vi "DepthSense Verbose Acquisition.vi"() -> ()   [LabVIEW 2011]
uses:
  <vilib>/vision/Image Controls.llb/IMAQ Image.ctl
  <vilib>/Platform/TimedLoop/XDataNode/timing_clust.ctl
  <vilib>/Platform/TimedLoop/XDataNode/nitl_modes.ctl
  <vilib>/Platform/TimedLoop/XDataNode/wakeup.ctl
  C:/Users/Behavior Room/Desktop/Kinect Mouse/DepthSense/FunctionPointerProxy/FunctionPointerProxy/bin/Release/FunctionPointerProxy.dll
  FunctionPointerProxy/FunctionPointerProxy/bin/Release/FunctionPointerProxy.dll
  IT WORKS SO SUCK IT/DepthSense Global Status.vi
  <vilib>/Platform/TimedLoop/XDataNode/XDataNode.xnode
  <userlib>/libOptrima-2-3/libOptrima-2-3.lvlib
  <vilib>/Platform/TimedLoop/XDataNode/XDNodeRunTimeDep.lvlib
  Program Files (x86)/SoftKinetic/OptrimaSDK/lib/libOptrima-2-3.dll
panel:
  out "Image":T1(plugin-control)
  out "Frame ID":i32
  in  "DepthSense Indicator":T2={"Camera Version"="", "Image Height"=0, "Image Width"=0, "Minimum Framerate"=0, "Maximum Framerate"=0, "Framerate"=25, "Close Mode"=FALSE, "Denoising"=FALSE, "Leakage Algorithm"=FALSE, "Anti-Aliasing"=FALSE, "Camera Status"=-2, "API Version"="", "Light Intensity"=100, "Confidence Threshold"=100, "Range"=0.0}
  in  "stop":bool
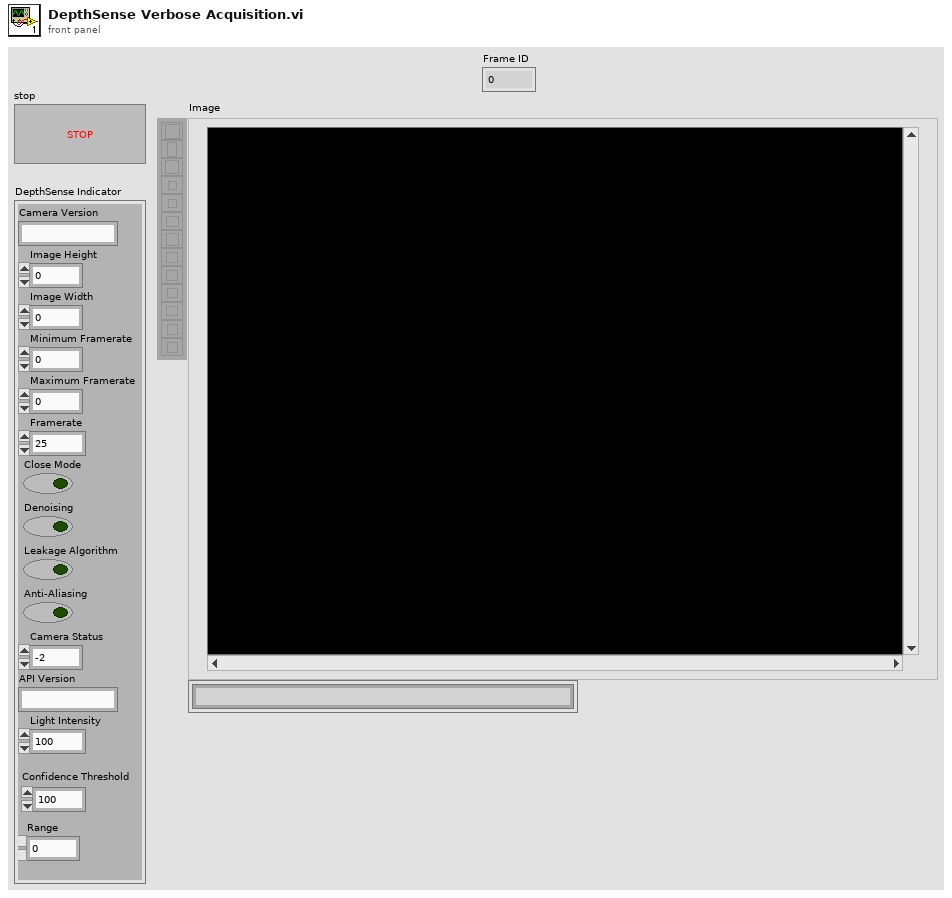
[diagram p1: front panel]
types:
  T1 = typedef "IMAQ Image.ctl" = refnum<image>
  T2 = cluster{"Camera Version":string, "Image Height":i32, "Image Width":i32, "Minimum Framerate":i32, "Maximum Framerate":i32, "Framerate":i32, "Close Mode":bool, "Denoising":bool, "Leakage Algorithm":bool, "Anti-Aliasing":bool, "Camera Status":i32, "API Version":string, "Light Intensity":i32, "Confidence Threshold":u16, "Range":dbl}
  T3 = cluster{"Camera Version":string, "Image Height":i32, "Image Width":i32, "Minimum Framerate":i32, "Maximum Framerate":i32, "Framerate":i32, "Close Mode":bool, "Denoising":bool, "Leakage Algorithm":bool, "Anti-Aliasing":bool, "Camera Status":i32, "API Version":string, "Light Intensity":i32, "Confidence Threshold":u16, "Range":sgl}
  T4 = typedef "t_CallbackReferences.ctl" = cluster{"LV event callback ":refnum<k27>, "Proxy instance":refnum<k24>, "(*f)(...)":i32}
  T5 = typedef "XDNodeRunTimeDep.lvlib/timing_clust.ctl" = cluster{"Expected End [f-1]":u64, "Actual End [f-1]":u64, "Finished Late? [f-1]":bool, "Expected End [i-1]":u64, "Actual End [i-1]":u64, "Finished Late? [i-1]":bool, "Expected Start [i]":u64, "Actual Start [i]":u64, "Expected Start [f]":u64, "Actual Start [f]":u64, "Source Name":string, "Structure Name":string, "Period":i64, "Deadline":i64, "Offset":i64, "Start":i64, "Priority":i32, "Timeout":i32, "Mode":T6, "Wakeup Reason":T7, "Error":errorcluster, "Source Type":string, "Secondary Source Type":string, "Global End Time":u64, "Global Start Time":u64, "Frame Duration":u64, "Iteration Duration":u64, "Assigned CPU":i32, "I/O Scan Engine Mode":u32}
  T6 = typedef "XDNodeRunTimeDep.lvlib/nitl_modes.ctl" = enum32{"No Change", "Process missed periods, maintain original phase", "Discard missed periods, maintain original phase", "Process missed periods, ignore original phase", "Discard missed periods, ignore original phase"}
  T7 = typedef "XDNodeRunTimeDep.lvlib/wakeup.ctl" = enum32{"Normal", "Aborted", "Asynchronous wakeup", "Timing source error", "Timed loop error", "Timeout"}
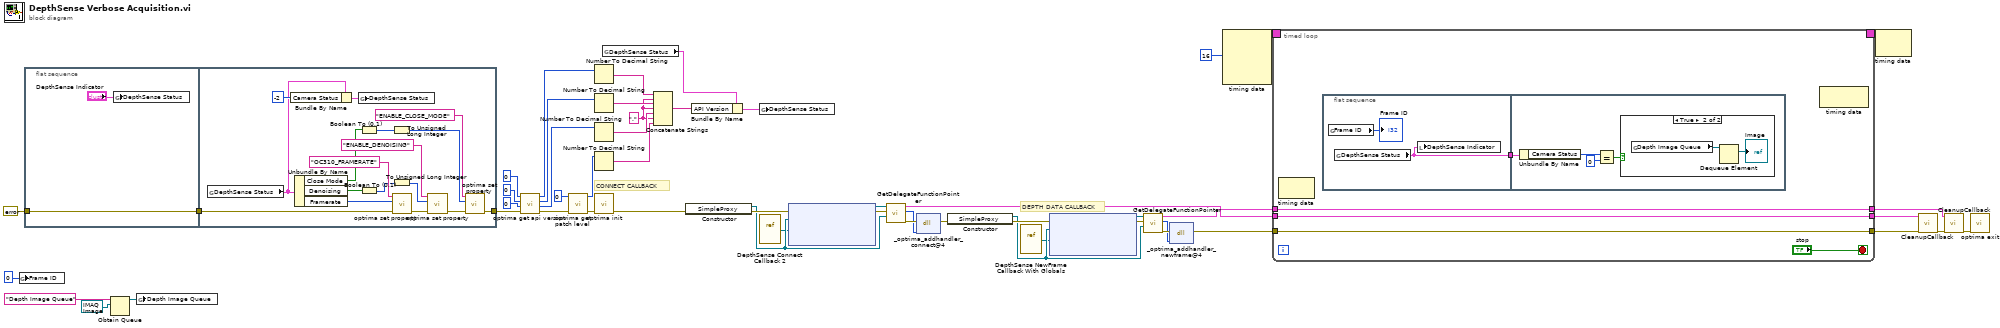
[diagram p0: block diagram]
diagram:
  w39 = "."
  # "DEPTH DATA CALLBACK"
  # "CONNECT CALLBACK"
  n1 = global write "DepthSense Global Status.vi" "Frame ID"(0 ("Frame ID")) -> ()
  n2 = flat-sequence {
    tunnel: errorcluster {"status"=FALSE, "code"=0, "source"=""} ("error in (no error)") -> [w54]
    tunnel: [w54] -> w1
    tunnel: [w69] -> w9
    tunnel: w1 -> [w63]
    frame #0 {
      n3 = global write "DepthSense Global Status.vi" "DepthSense Status"("DepthSense Indicator") -> ()
    }
    frame #1 {
      n4 = global read "DepthSense Global Status.vi" "DepthSense Status"() -> (w62:T3)
      n5 = Bundle By Name(cluster=w62, "Camera Status"=-2) -> (w71:T3)
      n6 = Unbundle By Name(w62) -> ("Close Mode"=w60:bool, "Denoising"=w58:bool, "Framerate"=w55:i32)
      n7 = global write "DepthSense Global Status.vi" "DepthSense Status"(w71) -> ()
      n8 = Boolean To (0,1)(Boolean=w60) -> (0, 1=w61:i16)
      n9 = Boolean To (0,1)(Boolean=w58) -> (0, 1=w59:i16)
      n10 = To Unsigned Long Integer(number=w61) -> (unsigned 32bit integer=w56:u32)
      n11 = To Unsigned Long Integer(number=w59) -> (unsigned 32bit integer=w57:u32)
      n12 = call <userlib>:"optrima set property.vi"("error in (no error)"=w63, "value"=w55, "name"="OC310_FRAMERATE") -> ("error out"=w66:errorcluster)  [unwired: 7 in, 1 out]
      n13 = call <userlib>:"optrima set property.vi"("error in (no error)"=w66, "value"=w57, "name"="ENABLE_DENOISING") -> ("error out"=w65:errorcluster)  [unwired: 7 in, 1 out]
      n14 = call <userlib>:"optrima set property.vi"("error in (no error)"=w65, "value"=w56, "name"="ENABLE_CLOSE_MODE") -> ("error out"=w69:errorcluster)  [unwired: 7 in, 1 out]
    }
  }
  n15 = Obtain Queue(name (unnamed)="Depth Image Queue", element data type=T1 refnum ("New Image")) -> (queue out=w28:refnum<queue>)  [unwired: 3 in, 2 out]
  n16 = global write "DepthSense Global Status.vi" "Depth Image Queue"(w28) -> ()
  n17 = call <userlib>:"optrima get api version.vi"("error in (no error)"=w9, "minor"=u32 0, "major"=u32 0, "release"=u32 0) -> ("error out"=w52:errorcluster, "minor out"=w49:u32, "major out"=w50:u32, "release out"=w51:u32)  [unwired: 4 in]
  n18 = call <userlib>:"optrima get patch level.vi"("error in (no error)"=w52, "patch"=u32 0) -> ("error out"=w8:errorcluster, "patch out"=w48:u32)  [unwired: 8 in]
  n19 = Number To Decimal String(number=w51) -> (decimal integer string=w47:string)  [unwired: 1 in]
  n20 = Number To Decimal String(number=w50) -> (decimal integer string=w42:string)  [unwired: 1 in]
  n21 = Number To Decimal String(number=w49) -> (decimal integer string=w41:string)  [unwired: 1 in]
  n22 = Number To Decimal String(number=w48) -> (decimal integer string=w40:string)  [unwired: 1 in]
  n23 = call <userlib>:"optrima init.vi"("error in (no error)"=w8) -> ("error out"=w7:errorcluster)  [unwired: 10 in]
  n24 = global read "DepthSense Global Status.vi" "DepthSense Status"() -> (w11:T3)
  n25 = Concatenate Strings(w47, w39, w42, w39, w41, w39, w40) -> (w31:string)
  n26 = constructor class="SimpleProxy"(error in=w7) -> (reference out=w35:refnum<k24>, error out=w38:errorcluster)  [unwired: 2 in, 1 out]
  n27 = Bundle By Name(cluster=w11, "API Version"=w31) -> (w12:T3)
  n28 = global write "DepthSense Global Status.vi" "DepthSense Status"(w12) -> ()
  n29 = vi-ref "DepthSense Connect Callback 2.vi"() -> ("vi reference"=w27:refnum<vi>)
  n30 = node(w38, w35, w27) -> (w37:refnum<k27>, w36:errorcluster)  [unwired: 2 in]
  n31 = call "GetDelegateFunctionPointer.vi"("target class"=w35, "error in (no error)"=w36, "event callback refnum"=w37) -> ("error out"=w34:errorcluster, "(*f)(...)"=w33:i32, "References"=w32:T4)  [unwired: 6 in]
  n32 = dll-call lib="C:/Program Files (x86)/SoftKinetic/OptrimaSDK/lib/libOptrima-2-3.dll" fn="_optrima_addhandler_connect@4"(error in=w34, "handlerfunc"=w33) -> (error out=w17:errorcluster)  [unwired: 4 in, 1 out]
  n33 = constructor class="SimpleProxy"(error in=w17) -> (reference out=w25:refnum<k24>, error out=w26:errorcluster)  [unwired: 2 in, 1 out]
  n34 = vi-ref "DepthSense NewFrame Callback With Globals.vi"() -> ("vi reference"=w20:refnum<vi>)
  n35 = node(w26, w25, w20) -> (w23:refnum<k27>, w24:errorcluster)  [unwired: 2 in]
  n36 = call "GetDelegateFunctionPointer.vi"("target class"=w25, "error in (no error)"=w24, "event callback refnum"=w23) -> ("error out"=w22:errorcluster, "(*f)(...)"=w21:i32, "References"=w19:T4)  [unwired: 6 in]
  n37 = dll-call lib="C:/Program Files (x86)/SoftKinetic/OptrimaSDK/lib/libOptrima-2-3.dll" fn="_optrima_addhandler_newframe@4"(error in=w22, "handlerfunc"=w21) -> (error out=w18:errorcluster)  [unwired: 4 in, 1 out]
  n38 = node-c288(i64 16 ("Period")) -> (w4:T5)  [unwired: 3 in]
  n39 = timed-loop {
    tunnel: [w76] -> w5
    tunnel: w18 -> [w76]
    tunnel: [w75] -> w14
    tunnel: w32 -> [w75]
    tunnel: w19 -> [w74]
    tunnel: [w74] -> w13
    timing: w4 -> [_]
    timing-out: [_] -> w3
    stop <- "stop" stop-if-true
    n40 = node-c288() -> ()  [unwired: 1 in, 1 out]
    n41 = flat-sequence {
      tunnel: [w80] -> w73
      tunnel: w73 -> [w81]
      frame #0 {
        n42 = global read "DepthSense Global Status.vi" "Frame ID"() -> (→"Frame ID":i32)
        n43 = global read "DepthSense Global Status.vi" "DepthSense Status"() -> (w80:T3)
        n44 = local write "DepthSense Indicator"(w80) -> ()
      }
      frame #1 {
        n45 = Unbundle By Name(w81) -> ("Camera Status"=w83:i32)
        n46 = Equal?(x=w83, y=0) -> (x = y?=w84:bool)
        n47 = case shown="True" w84 {
          frame False {
          }
          frame True {
            n48 = global read "DepthSense Global Status.vi" "Depth Image Queue"() -> (w86:refnum<queue>)
            n49 = Dequeue Element(queue=w86) -> (element=→"Image":T1)  [unwired: 2 in, 3 out]
          }
        }
      }
    }
    n50 = node-c288() -> ()  [unwired: 1 in, 1 out]
  }
  n51 = node-c288(w3) -> ()  [unwired: 1 out]
  n52 = call "CleanupCallback.vi"("error in (no error)"=w5, "References"=w14) -> ("error out"=w15:errorcluster)  [unwired: 9 in]
  n53 = call "CleanupCallback.vi"("error in (no error)"=w15, "References"=w13) -> ("error out"=w16:errorcluster)  [unwired: 9 in]
  n54 = call <userlib>:"optrima exit.vi"("error in (no error)"=w16) -> ()  [unwired: 10 in, 1 out]
